vi "Tick Quadrature State.vi"(7 "Forward? (T)":bool=TRUE, 8 "error in (no error)":errorcluster, 9 "Current State":i32, 10 "Channels":string[](array[string])=[" ", ""], 11 "WorkspaceManager in":T1) -> (0 "error out":errorcluster, 1 "New State":i32, 3 "WorkspaceManager out":T1)   [LabVIEW 2016, in "Scan Engine cRIO System Tests.lvclass"]
uses:
  Scan Engine cRIO System Tests.lvclass
  <vilib>/NI Veristand/Execution/Workspace/WorkspaceAPI.ctl
  NationalInstruments.VeriStand.ClientAPI
  <vilib>/NI Veristand/Execution/Workspace/NI VeriStand - Set Multiple Channel Values.vi
  <vilib>/NI VeriStand/Execution/Workspace/NI_VS Workspace ExecutionAPI.lvlib
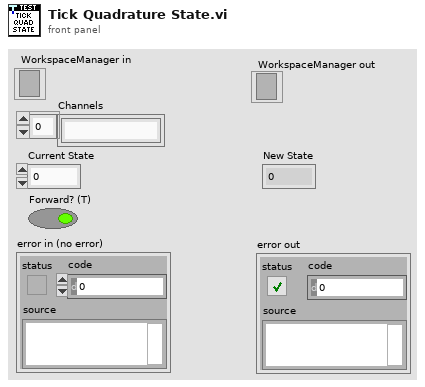
[diagram p1: front panel]
types:
  T1 = typedef "NI_VS Workspace ExecutionAPI.lvlib/WorkspaceAPI.ctl" = refnum<k24>
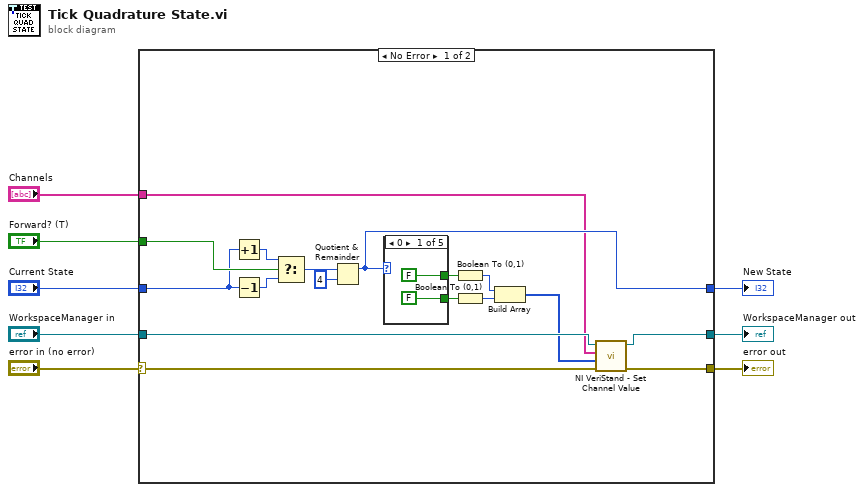
[diagram p0: block diagram]
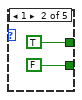
[diagram p2: hidden frame]
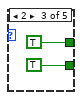
[diagram p3: hidden frame]
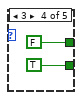
[diagram p4: hidden frame]
diagram:
  n1 = case shown="No Error" "error in (no error)" {
    selector: "error in (no error)" -> [w22 w36]
    tunnel: "Forward? (T)" -> [w25 _]
    tunnel: "WorkspaceManager in" -> [w24 w35]
    tunnel: [w23 w35] -> w6
    tunnel: [w21 w36] -> w4
    tunnel: [w11 w34] -> w1
    tunnel: "Channels" -> [w10 _]
    tunnel: "Current State" -> [w9 w34]
    frame No Error {
      n2 = Increment(x=w9) -> (x+1=w20:i32)
      n3 = Decrement(x=w9) -> (x-1=w19:i32)
      n4 = Select(t=w20, s=w25, f=w19) -> (s? t:f=w18:i32)
      n5 = Quotient & Remainder(x=w18, y=4) -> (x-y*floor(x/y)=w11:i32)  [unwired: 1 out]
      n6 = case shown="0" w11 {
        tunnel: [FALSE TRUE TRUE FALSE _] -> w16
        tunnel: [FALSE FALSE TRUE TRUE _] -> w15
        frame 0 {
        }
        frame 1 {
        }
        frame 2 {
        }
        frame 3 {
        }
        frame Default {
        }
      }
      n7 = Boolean To (0,1)(Boolean=w16) -> (0, 1=w14:i16)
      n8 = Boolean To (0,1)(Boolean=w15) -> (0, 1=w13:i16)
      n9 = Build Array(w14, w13) -> (w12:i16[])
      n10 = call-poly <vilib>:"NI VeriStand - Set Channel Value.vi"("error in (no error)"=w22, "Values"=w12, "Channels"=w10, "WorkspaceManager in"=w24) -> ("error out"=w21:errorcluster, "WorkspaceManager out"=w23:T1)  [unwired: 6 in]
    }
    frame Error {
    }
  }
  "WorkspaceManager out" <- w6
  "error out" <- w4
  "New State" <- w1
